vi "Launch_Dialog.vi"(8 "error in (no error)":errorcluster, 10 "Dialog Text In":variant) -> (0 "error out":errorcluster)   [LabVIEW 2019, in "MHL.lvlib"]
uses:
  MHL.lvlib
  typedef/MHL_Data.ctl
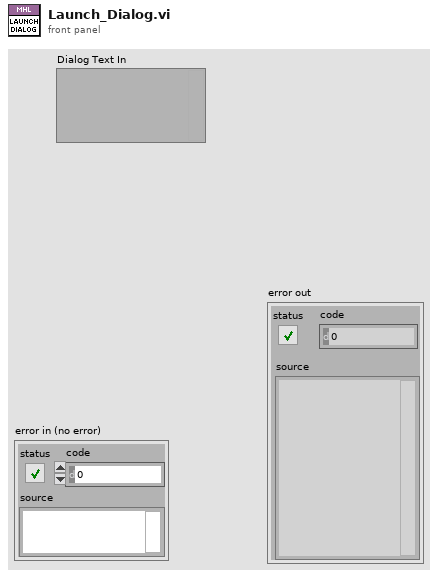
[diagram p1: front panel]
types:
  T1 = typedef "MHL.lvlib/MHL_Data.ctl" = cluster{"Ctrl_Refs":cluster{"Quit":refnum<vi>, "Motor_Switch":refnum<vi>, "Status":refnum<vi>, "Alarm_Panel":refnum<vi>, "Bearing Temp Chart":refnum<vi>, "Motor Temp Chart":refnum<vi>, "TabCtl":refnum<vi>, "Bearing Temp Clust":refnum<vi>}, "Main_Ref":refnum<vi>}
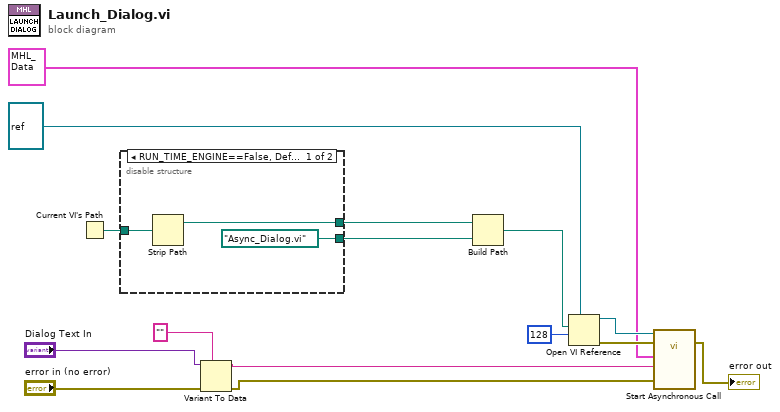
[diagram p0: block diagram]
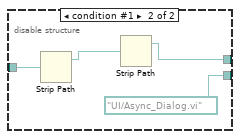
[diagram p2: hidden frame]
diagram:
  n1 = Current VI's Path() -> (path=w8:path)
  n2 = disable-structure shown="RUN_TIME_ENGINE==False, Default" {
    disable-tunnel: w8 -> [w18 w22]
    disable-tunnel: [w17 w20] -> w7
    disable-tunnel: [path "Async_Dialog.vi" path "UI/Async_Dialog.vi"] -> w6
    frame condition #0 (active) {
      n3 = Strip Path(path=w18) -> (stripped path=w17:path)  [unwired: 1 out]
    }
    frame condition #1 {
      n4 = Strip Path(path=w22) -> (stripped path=w21:path)  [unwired: 1 out]
      n5 = Strip Path(path=w21) -> (stripped path=w20:path)  [unwired: 1 out]
    }
  }
  n6 = Variant To Data(error in="error in (no error)", type="", Variant="Dialog Text In") -> (data=w2:string, error out=w1:errorcluster)
  n7 = Build Path(base path=w7, name or relative path=w6) -> (appended path=w10:path)
  n8 = Open VI Reference(type specifier VI Refnum (for type only)=refnum<vi> refnum, vi path=w10, options=128) -> (vi reference=w14:refnum<vi>, error out=w13:errorcluster)  [unwired: 3 in]
  n9 = call-by-ref "Start Asynchronous Call"(reference=w14, error in=w13, 8:"error in (no error)"=w1, "Dialog Text In"=w2, "MHL_Data"=T1 {"Ctrl_Refs"={"Quit"=refnum, "Motor_Switch"=refnum, "Status"=refnum, "Alarm_Panel"=refnum, "Bearing Temp Chart"=refnum, "Motor Temp Chart"=refnum, "TabCtl"=refnum, "Bearing Temp Clust"=refnum}, "Main_Ref"=refnum}) -> (error out=→"error out":errorcluster)  [unwired: 7 in, 3 out]
